vi "KalmanFilter_GetK_Single.vi"(9 "Column":i32, 10 "Row":i32, 11 "in KalmanFilter":T1) -> (3 "K":dbl)   [LabVIEW 2019, in "Trajectory_Library.lvlib"]
doc: "Creates a new LINEAR SYSTEM data cluster with the specified values. \n\n\nInputs: \n - XXX -- XXX.\n\nOutputs:\n - XXX -- XXX."
uses:
  KALMAN_FILTER.ctl
  <vilib>/Analysis/Matrix/Datatypes/RealMatrix.ctl
  LINEAR_SYSTEM.ctl
  Trajectory_Library.lvlib
  <vilib>/Analysis/Matrix/NI_Matrix.lvlib
panel:
  # "Steady State Gain  \n<States,Outputs>"
  # "State Estimate <Statess,1>"
  # "<States,States>"
  # "<States,Inputs>"
  # "<Outputs,States>"
  # "<Outputs,Inputs>"
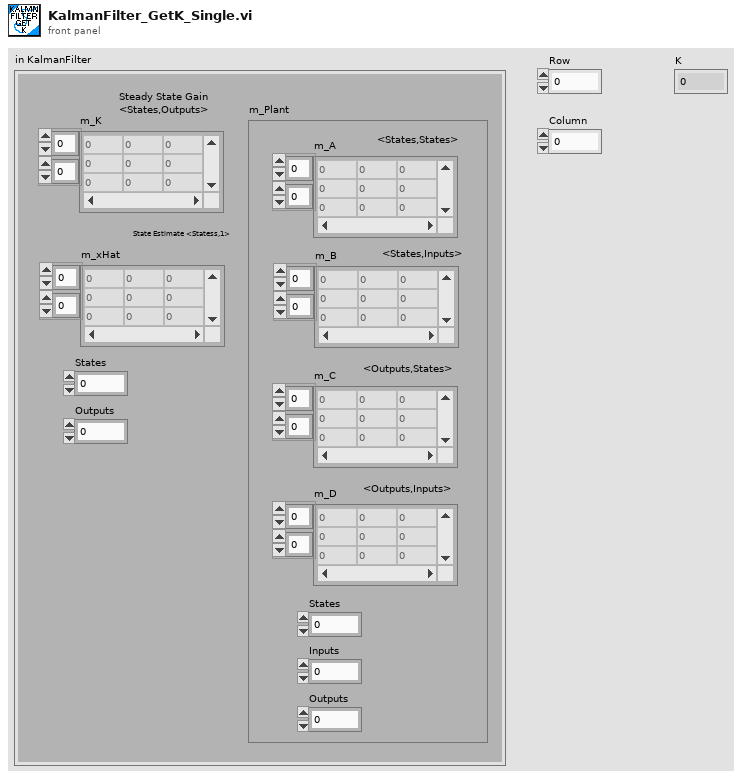
[diagram p1: front panel]
types:
  T1 = typedef "Trajectory_Library.lvlib/KALMAN_FILTER.ctl" = cluster{"m_K":T2, "m_xHat":T2, "States":i32, "Outputs":i32, "m_Plant":T3}
  T2 = typedef "NI_Matrix.lvlib/RealMatrix.ctl" = dbl[][]
  T3 = typedef "Trajectory_Library.lvlib/LINEAR_SYSTEM.ctl" = cluster{"m_A":T2, "m_B":T2, "m_C":T2, "m_D":T2, "States":i32, "Inputs":i32, "Outputs":i32}
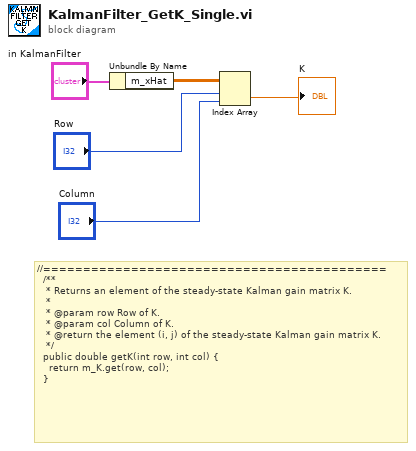
[diagram p0: block diagram]
diagram:
  # "//===========================================\n  /**\n   * Returns an element of the steady-state Kalman gain matrix K.\n   *\n   * @param row Row of K.\n   * @param col Column of K.\n   * @return the element (i, j) of the steady-state Kalman gain matrix K.\n   */\n  public double getK(int row, int col) {\n    return m_K.get(row, col);\n  }"
  n1 = Unbundle By Name("in KalmanFilter") -> ("m_xHat"=w4:T2)
  n2 = Index Array(array=w4, index (row)="Row", index (col)="Column") -> (element=→"K":dbl)
